vi "Tree Value Change.vi"(10 "Tree Data":cluster{"Tag":string[], "Settings":T1[]} {"Settings"."Data Type" items=["Tree Parent"=-1, "Numeric"=0, "String"=1, "Boolean"=2, "Enum"=3]}, 11 "Init Refs":T3) -> (3 "Value":string)   [LabVIEW 2020, in "Sequencer with Output Values.lvlib" / "Sequencer with Output Values.lvclass"]
uses:
  Sequencer with Output Values.lvclass
  Control Refs.ctl
  Tree Item Settings.ctl
  Data Type.ctl
  <vilib>/Utility/miscctls.llb/LVPositionTypeDef.ctl
  Data Type Enum.ctl
  Global Tree Data.vi
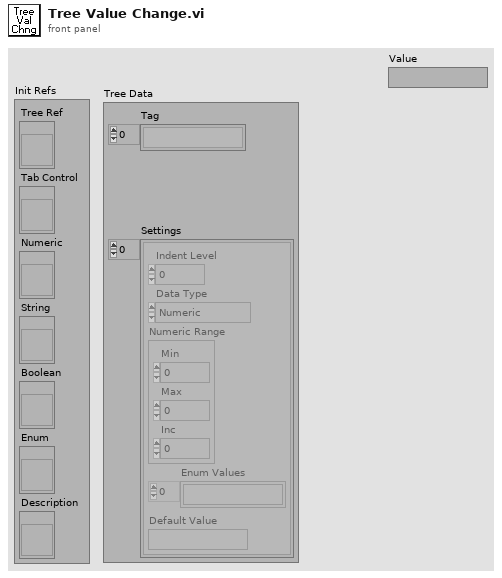
[diagram p1: front panel]
types:
  T1 = typedef "Sequencer with Output Values.lvlib/Sequencer with Output Values.lvclass/Tree Item Settings.ctl" = cluster{"Indent Level":i32, "Data Type":T2, "Numeric Range":cluster{"Min":dbl, "Max":dbl, "Inc":dbl}, "Enum Values":string[], "Default Value":string}
  T2 = typedef "Sequencer with Output Values.lvlib/Sequencer with Output Values.lvclass/Data Type.ctl" = i16
  T3 = typedef "Sequencer with Output Values.lvlib/Sequencer with Output Values.lvclass/Control Refs.ctl" = cluster{"Tree Ref":refnum<vi>, "Tab Control":refnum<vi>, "Numeric":refnum<vi>, "String":refnum<vi>, "Boolean":refnum<vi>, "Enum":refnum<vi>, "Description":refnum<vi>}
  T4 = typedef "LVPositionTypeDef.ctl" = cluster{"Left":i32, "Top":i32}
  T5 = typedef "Sequencer with Output Values.lvlib/Sequencer with Output Values.lvclass/Data Type Enum.ctl" = enum16{"Numeric", "String", "Boolean", "Enum"}
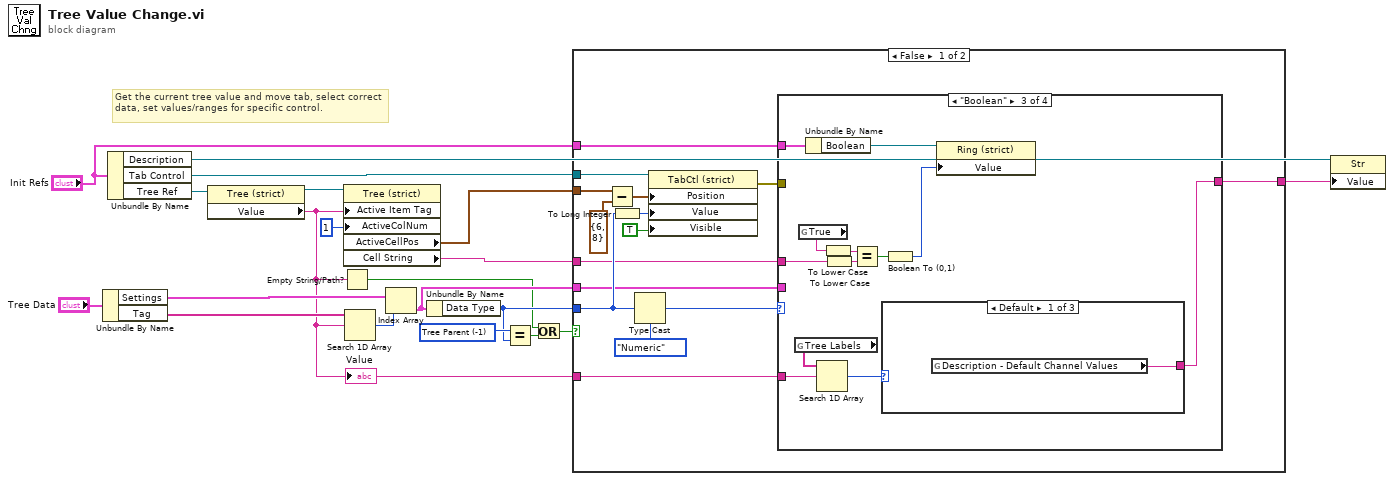
[diagram p0: block diagram]
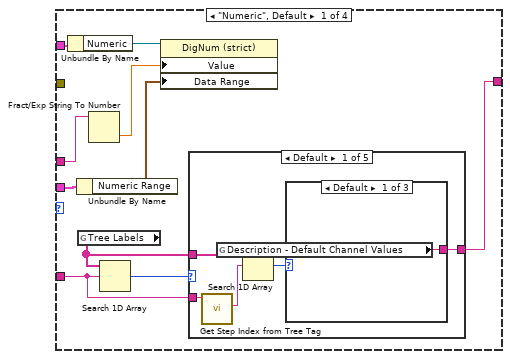
[diagram p2: hidden frame]
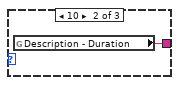
[diagram p3: hidden frame]
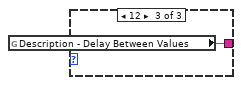
[diagram p4: hidden frame]
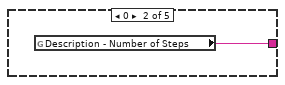
[diagram p5: hidden frame]
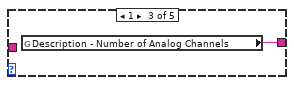
[diagram p6: hidden frame]
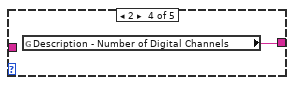
[diagram p7: hidden frame]
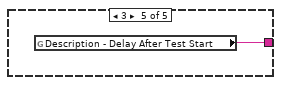
[diagram p8: hidden frame]
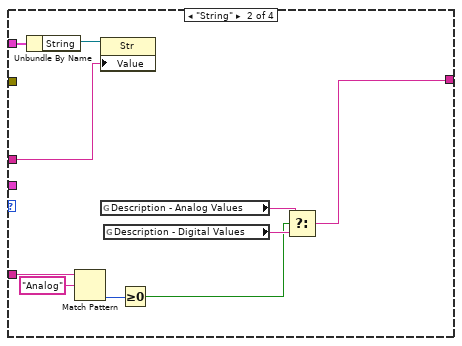
[diagram p9: hidden frame]
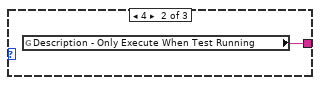
[diagram p10: hidden frame]
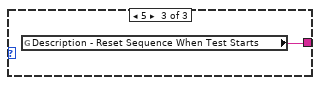
[diagram p11: hidden frame]
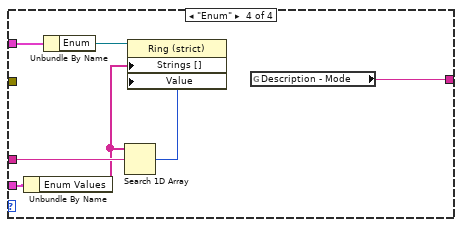
[diagram p12: hidden frame]
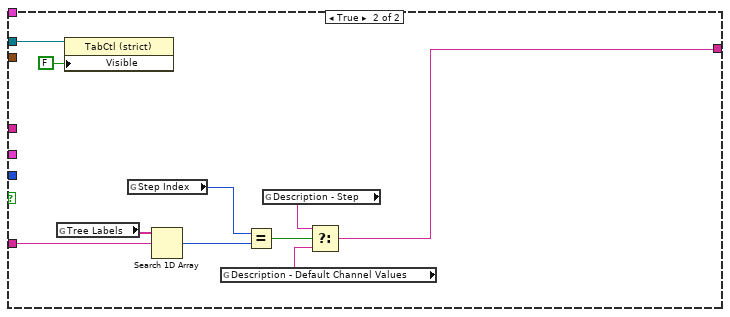
[diagram p13: hidden frame]
diagram:
  w11 = T2 -1 items=["Tree Parent"=-1, "Numeric"=0, "String"=1, "Boolean"=2, "Enum"=3, "Command"=4, "Numeric Min/Max"=5] ("Data Type")
  # "Get the current tree value and move tab, select correct data, set values/ranges for specific control."
  n1 = Unbundle By Name("Tree Data") -> ("Settings"=w13:T1[], "Tag"=w14:string[])
  n2 = Unbundle By Name("Init Refs") -> ("Description"=w3:refnum<vi>, "Tab Control"=w17:refnum<vi>, "Tree Ref"=w20:refnum<vi>)
  n3 = property class="Tree (strict)"(reference=w20) -> (reference out=w19:refnum<vi>, "Value"=w1:string)  [unwired: 1 in, 1 out]
  "Value" <- w1
  n4 = Empty String/Path?(string/path=w1) -> (empty?=w5:bool)
  n5 = property class="Tree (strict)"(reference=w19, "Active Item Tag"=w1, "ActiveColNum"=1 ("Active Cell:Active Column Number")) -> ("ActiveCellPos"=w16:T4, "Cell String"=w9:string)  [unwired: 1 in, 2 out]
  n6 = Search 1D Array(1D array=w14, element=w1) -> (index of element=w12:i32)  [unwired: 1 in]
  n7 = Index Array(array=w13, index=w12) -> (element=w8:T1)
  n8 = Unbundle By Name(w8) -> ("Data Type"=w7:T2)
  n9 = Equal?(x=w11, y=w7) -> (x = y?=w6:bool)
  n10 = Or(x=w5, y=w6) -> (x .or. y?=w4:bool)
  n11 = case shown="False" w4 {
    tunnel: w17 -> [w35 w99]
    tunnel: w16 -> [w32 _]
    tunnel: w7 -> [w29 _]
    tunnel: "Init Refs" -> [w25 _]
    tunnel: w9 -> [w24 _]
    tunnel: w8 -> [w23 _]
    tunnel: [w22 w90] -> w2
    tunnel: w1 -> [w21 w96]
    frame False {
      n12 = Subtract(x=w32, y=T4 {"Left"=6, "Top"=8}) -> (x-y=w31:T4)
      n13 = To Long Integer(number=w29) -> (32bit integer=w34:i32)
      n14 = Type Cast(type=Data_Type_Enum."Numeric" ("Data Type"), x=w29) -> (*(type *) &x=w27:T5)
      n15 = property class="TabCtl (strict)"(reference=w35, "Position"=w31, "Value"=w34, "Visible"=TRUE) -> (error out=w26:errorcluster)  [unwired: 1 in, 1 out]
      n16 = case shown="\"Boolean\"" w27 {
        tunnel: w26 -> [_ _ _ _]
        tunnel: w25 -> [w45 w67 w79 w89]
        tunnel: w24 -> [w42 w65 w77 w86]
        tunnel: w23 -> [w43 _ _ w87]
        tunnel: [w38 w58 w68 w83] -> w22
        tunnel: w21 -> [w37 w62 w70 _]
        frame "Numeric", Default {
          n17 = Unbundle By Name(w45) -> ("Numeric"=w44:refnum<vi>)
          n18 = Unbundle By Name(w43) -> ("Numeric Range"=w40:cluster{"Min":dbl, "Max":dbl, "Inc":dbl})
          n19 = global read "Global Tree Data.vi" "Tree Labels"() -> (w36:string[])
          n20 = Fract/Exp String To Number(string=w42) -> (number=w41:dbl)  [unwired: 3 in, 1 out]
          n21 = Search 1D Array(1D array=w36, element=w37) -> (index of element=w39:i32)  [unwired: 1 in]
          n22 = property class="DigNum (strict)"(reference=w44, "Value"=w41, "Data Range"=w40) -> ()  [unwired: 1 in, 2 out]
          n23 = case shown="Default" w39 {
            tunnel: [w46 w54 w55 w56 w57] -> w38
            tunnel: w37 -> [w50 _ _ _ _]
            tunnel: w36 -> [w49 _ _ _ _]
            frame Default {
              n24 = call "Get Step Index from Tree Tag.vi"("Tree Tag"=w50) -> ("Step Param String"=w48:string)  [unwired: 9 in, 1 out]
              n25 = Search 1D Array(1D array=w49, element=w48) -> (index of element=w47:i32)  [unwired: 1 in]
              n26 = case shown="Default" w47 {
                tunnel: [w51 w52 w53] -> w46
                frame Default {
                  n27 = global read "Global Tree Data.vi" "Description - Default Channel Values"() -> (w51:string)
                }
                frame 10 {
                  n28 = global read "Global Tree Data.vi" "Description - Duration"() -> (w52:string)
                }
                frame 12 {
                  n29 = global read "Global Tree Data.vi" "Description - Delay Between Values"() -> (w53:string)
                }
              }
            }
            frame 0 {
              n30 = global read "Global Tree Data.vi" "Description - Number of Steps"() -> (w54:string)
            }
            frame 1 {
              n31 = global read "Global Tree Data.vi" "Description - Number of Analog Channels"() -> (w55:string)
            }
            frame 2 {
              n32 = global read "Global Tree Data.vi" "Description - Number of Digital Channels"() -> (w56:string)
            }
            frame 3 {
              n33 = global read "Global Tree Data.vi" "Description - Delay After Test Start"() -> (w57:string)
            }
          }
        }
        frame "String" {
          n34 = Unbundle By Name(w67) -> ("String"=w66:refnum<vi>)
          n35 = Match Pattern(string=w62, regular expression="Analog") -> (offset past match=w60:i32)  [unwired: 1 in, 3 out]
          n36 = property class="Str"(reference=w66, "Value"=w65) -> ()  [unwired: 1 in, 2 out]
          n37 = global read "Global Tree Data.vi" "Description - Analog Values"() -> (w64:string)
          n38 = global read "Global Tree Data.vi" "Description - Digital Values"() -> (w63:string)
          n39 = Greater Or Equal To 0?(x=w60) -> (x >= 0?=w59:bool)
          n40 = Select(t=w64, s=w59, f=w63) -> (s? t:f=w58:string)
        }
        frame "Boolean" {
          n41 = global read "Global Tree Data.vi" "Tree Labels"() -> (w71:string[])
          n42 = global read "Global Tree Data.vi" "True"() -> (w73:string)
          n43 = Unbundle By Name(w79) -> ("Boolean"=w78:refnum<vi>)
          n44 = Search 1D Array(1D array=w71, element=w70) -> (index of element=w69:i32)  [unwired: 1 in]
          n45 = To Lower Case(string=w73) -> (all lower case string=w72:string)
          n46 = To Lower Case(string=w77) -> (all lower case string=w76:string)
          n47 = Equal?(x=w72, y=w76) -> (x = y?=w75:bool)
          n48 = case shown="Default" w69 {
            tunnel: [w80 w81 w82] -> w68
            frame Default {
              n49 = global read "Global Tree Data.vi" "Description - Default Channel Values"() -> (w80:string)
            }
            frame 4 {
              n50 = global read "Global Tree Data.vi" "Description - Only Execute When Test Running"() -> (w81:string)
            }
            frame 5 {
              n51 = global read "Global Tree Data.vi" "Description - Reset Sequence When Test Starts"() -> (w82:string)
            }
          }
          n52 = Boolean To (0,1)(Boolean=w75) -> (0, 1=w74:i16)
          n53 = property class="Ring (strict)"(reference=w78, "Value"=w74) -> ()  [unwired: 1 in, 2 out]
        }
        frame "Enum" {
          n54 = Unbundle By Name(w87) -> ("Enum Values"=w85:string[])
          n55 = Unbundle By Name(w89) -> ("Enum"=w88:refnum<vi>)
          n56 = Search 1D Array(1D array=w85, element=w86) -> (index of element=w84:i32)  [unwired: 1 in]
          n57 = property class="Ring (strict)"(reference=w88, "Strings []"=w85, "Value"=w84) -> ()  [unwired: 1 in, 2 out]
          n58 = global read "Global Tree Data.vi" "Description - Mode"() -> (w83:string)
        }
      }
    }
    frame True {
      n59 = global read "Global Tree Data.vi" "Tree Labels"() -> (w97:string[])
      n60 = property class="TabCtl (strict)"(reference=w99, "Visible"=FALSE) -> ()  [unwired: 1 in, 2 out]
      n61 = global read "Global Tree Data.vi" "Step Index"() -> (w94:i32)
      n62 = Search 1D Array(1D array=w97, element=w96) -> (index of element=w95:i32)  [unwired: 1 in]
      n63 = global read "Global Tree Data.vi" "Description - Default Channel Values"() -> (w91:string)
      n64 = Equal?(x=w94, y=w95) -> (x = y?=w93:bool)
      n65 = global read "Global Tree Data.vi" "Description - Step"() -> (w92:string)
      n66 = Select(t=w92, s=w93, f=w91) -> (s? t:f=w90:string)
    }
  }
  n67 = property class="Str"(reference=w3, "Value"=w2) -> ()  [unwired: 1 in, 2 out]
